vi "2Slave.vi"(8 "error in (no error)":errorcluster, 10 "Stop Ref":refnum<vi>) -> (0 "error out":errorcluster)   [LabVIEW 2014]
panel:
  out "error out 2":errorcluster
  out "Value":bool
  out "i":i32
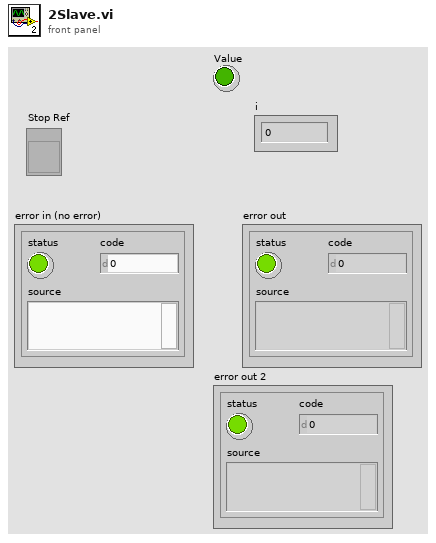
[diagram p1: front panel]
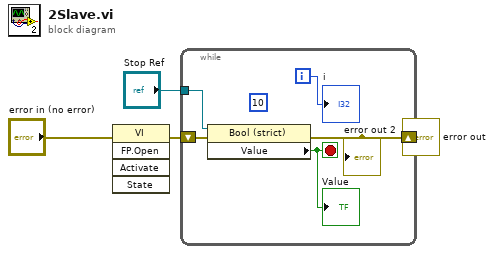
[diagram p0: block diagram]
diagram:
  n1 = invoke class="VI" method="FP.Open"(error in="error in (no error)") -> (error out=w1:errorcluster)  [unwired: 4 in, 4 out]
  n2 = while {
    tunnel: "Stop Ref" -> [w8]
    shift-right: [w5] -> w3
    shift-left: w1 -> [w6]
    i -> [w9]
    stop <- w7 stop-if-true
    (unwired) 10
    n3 = property class="Bool (strict)"(reference=w8, error in=w6) -> (error out=w5:errorcluster, "Value"=w7:bool)  [unwired: 1 out]
    "Value" <- w7
    "error out 2" <- w5
    "i" <- w9
  }
  "error out" <- w3
